vi "fpga_LP2 Filter_multunit0 (M Class_50Hz).vi"(0 "opState":T1, 2 "x":fxp<+/-,32,5>, 3 "coef":fxp<+/-,19,-3>) -> (4 "x(n-1)":fxp<+/-,32,5>, 7 "y":fxp<+/-,48,6>)   [LabVIEW 2013, in "NI_EP_PMU_FPGA.lvlib"]
uses:
  <vilib>/addons/Electrical Power/PMU/NI_EP_PMU_FPGA.lvlib
  <vilib>/rvi/Emulation/niFpgaSctlEmulationGetInTimedLoop.vi
  <vilib>/rvi/DataTransferAndStorage/Container/Common/niFpgaContainerGetUniqueNameForEmu.vi
  <vilib>/rvi/DataTransferAndStorage/Container/Common/niFpgaContainerSetEmuInfo.vi
  <vilib>/rvi/eio/common/nirviEmuReportErrorAndStop.vi
  <vilib>/rvi/Memory/Memory_Emulation/nirvimemoryEmulation.vi
  <vilib>/rvi/Memory/Memory_Emulation/nirvimemoryFastEmulation.vi
  <vilib>/rvi/Memory/Memory_Emulation/niFpgaMemoryEmulationCacheClearOnFirstRun.vi
  <vilib>/rvi/Memory/Memory_Emulation/nirvimemoryEmulationManagerCache_MakeExclusive.vi
  <vilib>/rvi/Memory/Memory_Emulation/niFpgaMemoryEmulationValidateCache.vi
  <vilib>/rvi/Memory/Memory_Emulation/nirvimemoryEmulationManagerCache_ReleaseExclusive.vi
  <vilib>/rvi/Memory/Memory_Emulation/nirvimemoryEmulationManagerCache_InsertValue.vi
  <vilib>/Utility/error.llb/Clear Errors.vi
  <vilib>/rvi/Memory/Memory_Emulation/nirvimemoryEmulationManagerCache_GetValue.vi
  <vilib>/rvi/Memory/Memory_Emulation/nirvimemoryEmulationManagerCache_SetValue.vi
  <vilib>/rvi/Emulation/niFpgaSctlEmulationResourceMgr.vi
  <vilib>/rvi/LocalResourceManager/LocalResourceManager.xnode
  <vilib>/rvi/DataTransferAndStorage/Container/XNode/niFpgaContainer.xnode
  <vilib>/rvi/FXPMathLib/FxpMul/XNode/nifxpmath_Multiplier.xnode
  <vilib>/rvi/FXPMathLib/sim/FxpSim.dll
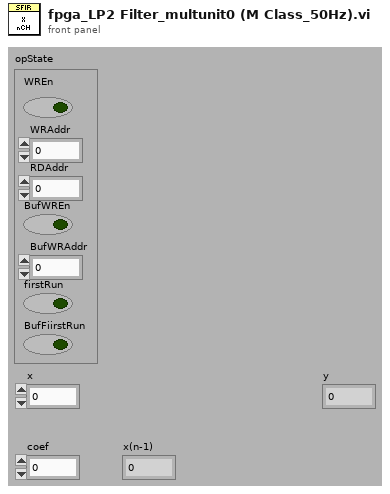
[diagram p1: front panel]
types:
  T1 = cluster{"WREn":bool, "WRAddr":fxp<+,14,14>, "RDAddr":fxp<+,14,14>, "BufWREn":bool, "BufWRAddr":fxp<+,14,14>, "firstRun":bool, "BufFiirstRun":bool}
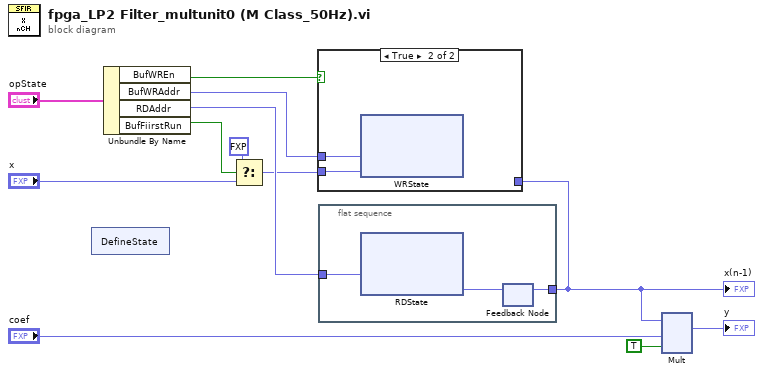
[diagram p0: block diagram]
diagram:
  n1 = xnode ("DefineState")() -> ()  [unwired: 1 out]
  n2 = Unbundle By Name("opState") -> ("BufWREn"=w8:bool, "BufWRAddr"=w7:fxp<+,14,14>, "RDAddr"=w9:fxp<+,14,14>, "BufFiirstRun"=w5:bool)
  n3 = Select(t=fxp<+/-,32,5> 0.0 ("zero"), s=w5, f="x") -> (s? t:f=w3:fxp<+/-,32,5>)
  n4 = case shown="True" w8 {
    tunnel: w3 -> [_ w14]
    tunnel: w7 -> [_ w13]
    tunnel: w1 -> [_ _]
    frame False {
    }
    frame True {
      n5 = xnode ("WRState")("Address"=w13, "Data"=w14) -> ()  [unwired: 1 in, 1 out]
    }
  }
  n6 = flat-sequence {
    tunnel: [w17] -> w1
    tunnel: w9 -> [w15]
    frame #0 {
      n7 = xnode ("RDState")("Address"=w15) -> ("Data"=w16:fxp<+/-,32,5>)  [unwired: 1 in, 1 out]
      n8 = feedback-in #1(w16) -> ()
      n9 = feedback #1() -> (w17:fxp<+/-,32,5>)  [unwired: 1 out]
    }
  }
  n10 = xnode ("Mult")("x"=w1, "y"="coef", "input valid"=TRUE) -> ("x*y"=→"y":fxp<+/-,48,6>)  [unwired: 1 in, 2 out]
  "x(n-1)" <- w1
